vi "Read.vi"(8 "error in":errorcluster, 11 "Cycler Cluster - 24 Channel.lvclass":refnum<class "Cycler Cluster - 24 Channel.lvclass">) -> (0 "error out":errorcluster, 3 "output cluster":refnum<class "Cycler Cluster - 24 Channel.lvclass">)   [LabVIEW 2023, in "Cycler Cluster - 24 Channel.lvclass"]
uses:
  Cycler Cluster - 24 Channel.lvclass
  Cycler Cluster - 24 Channel.lvclass/Cycler Cluster - 24 Channel.ctl
  63f58f61-d796-4b25-88da-0470b2e22bf3.vi
  00f2480c-82fd-4dbd-adb2-7db79231ca1c.vi
  a45d338c-933b-4179-9ec5-1bb175e221a9.vi
  3e7895c2-778d-41f3-8bcc-0a004ba5d0e6.vi
  a5f17dcd-adde-4f08-8f4e-8c8580528fc1.vi
  ed9361c3-689c-4e9b-add1-8b87589797f0.vi
  6a4160ad-b9eb-4b5d-957b-ca1972af427b.vi
  340e8093-4c33-452f-a0fc-ec0f0c816548.vi
  4acc0959-a97e-40d2-905f-e4b53c5396e1.vi
  9ce8a87f-1424-40f7-aba3-ebfca12f9530.vi
  db8316ad-a1f6-46f4-a9d7-3ff13c7a6c53.vi
  3280034d-1119-4562-8431-d6c79152f843.vi
  5cec743d-8e0c-44d6-a509-ac96f90befc9.vi
  f015e34a-d19a-4af2-9a20-24b0ffa0b5d3.vi
  0afebac1-deb8-4dea-a382-2e4262eb9ab7.vi
  1ba67a8f-3263-44e6-b47e-6b1f46c6cf02.vi
  71f8bbf1-da11-439f-874e-3e528bdfa749.vi
  0c8128a7-c07e-44cb-ab87-c3f617b7e890.vi
  e505fce4-1dbe-4dbd-969b-5f8f6cb92da5.vi
  110d711f-602d-45bb-9c3c-bc18ca51752e.vi
  a3c512e7-962e-4a93-8488-56a803890fdd.vi
  4f6d0910-25e4-400a-b4c5-092e8cc88d34.vi
  4448cff9-e18d-4a6b-945e-10b1e3fd2828.vi
  4a46be96-aeb5-43b7-9243-adca9a8444cf.vi
  27230f32-3038-432e-846c-8983fd03581f.vi
  63f58f61-d796-4b25-88da-0470b2e22bf3.vi/c28b0ead-42ad-4072-80a2-aca7f2bd7ce3.vi
  63f58f61-d796-4b25-88da-0470b2e22bf3.vi/219d0231-d98b-4193-b5cc-84f90e3c9091.vi
  00f2480c-82fd-4dbd-adb2-7db79231ca1c.vi/c28b0ead-42ad-4072-80a2-aca7f2bd7ce3.vi
  00f2480c-82fd-4dbd-adb2-7db79231ca1c.vi/219d0231-d98b-4193-b5cc-84f90e3c9091.vi
  a45d338c-933b-4179-9ec5-1bb175e221a9.vi/c28b0ead-42ad-4072-80a2-aca7f2bd7ce3.vi
  a45d338c-933b-4179-9ec5-1bb175e221a9.vi/219d0231-d98b-4193-b5cc-84f90e3c9091.vi
  3e7895c2-778d-41f3-8bcc-0a004ba5d0e6.vi/c28b0ead-42ad-4072-80a2-aca7f2bd7ce3.vi
  3e7895c2-778d-41f3-8bcc-0a004ba5d0e6.vi/219d0231-d98b-4193-b5cc-84f90e3c9091.vi
  a5f17dcd-adde-4f08-8f4e-8c8580528fc1.vi/c28b0ead-42ad-4072-80a2-aca7f2bd7ce3.vi
  a5f17dcd-adde-4f08-8f4e-8c8580528fc1.vi/219d0231-d98b-4193-b5cc-84f90e3c9091.vi
  ed9361c3-689c-4e9b-add1-8b87589797f0.vi/c28b0ead-42ad-4072-80a2-aca7f2bd7ce3.vi
  ed9361c3-689c-4e9b-add1-8b87589797f0.vi/219d0231-d98b-4193-b5cc-84f90e3c9091.vi
  6a4160ad-b9eb-4b5d-957b-ca1972af427b.vi/c28b0ead-42ad-4072-80a2-aca7f2bd7ce3.vi
  6a4160ad-b9eb-4b5d-957b-ca1972af427b.vi/219d0231-d98b-4193-b5cc-84f90e3c9091.vi
  340e8093-4c33-452f-a0fc-ec0f0c816548.vi/c28b0ead-42ad-4072-80a2-aca7f2bd7ce3.vi
  340e8093-4c33-452f-a0fc-ec0f0c816548.vi/219d0231-d98b-4193-b5cc-84f90e3c9091.vi
  4acc0959-a97e-40d2-905f-e4b53c5396e1.vi/c28b0ead-42ad-4072-80a2-aca7f2bd7ce3.vi
  4acc0959-a97e-40d2-905f-e4b53c5396e1.vi/219d0231-d98b-4193-b5cc-84f90e3c9091.vi
  9ce8a87f-1424-40f7-aba3-ebfca12f9530.vi/c28b0ead-42ad-4072-80a2-aca7f2bd7ce3.vi
  9ce8a87f-1424-40f7-aba3-ebfca12f9530.vi/219d0231-d98b-4193-b5cc-84f90e3c9091.vi
  db8316ad-a1f6-46f4-a9d7-3ff13c7a6c53.vi/c28b0ead-42ad-4072-80a2-aca7f2bd7ce3.vi
  db8316ad-a1f6-46f4-a9d7-3ff13c7a6c53.vi/219d0231-d98b-4193-b5cc-84f90e3c9091.vi
  3280034d-1119-4562-8431-d6c79152f843.vi/c28b0ead-42ad-4072-80a2-aca7f2bd7ce3.vi
  3280034d-1119-4562-8431-d6c79152f843.vi/219d0231-d98b-4193-b5cc-84f90e3c9091.vi
  5cec743d-8e0c-44d6-a509-ac96f90befc9.vi/c28b0ead-42ad-4072-80a2-aca7f2bd7ce3.vi
  5cec743d-8e0c-44d6-a509-ac96f90befc9.vi/219d0231-d98b-4193-b5cc-84f90e3c9091.vi
  f015e34a-d19a-4af2-9a20-24b0ffa0b5d3.vi/c28b0ead-42ad-4072-80a2-aca7f2bd7ce3.vi
  f015e34a-d19a-4af2-9a20-24b0ffa0b5d3.vi/219d0231-d98b-4193-b5cc-84f90e3c9091.vi
  0afebac1-deb8-4dea-a382-2e4262eb9ab7.vi/c28b0ead-42ad-4072-80a2-aca7f2bd7ce3.vi
  0afebac1-deb8-4dea-a382-2e4262eb9ab7.vi/219d0231-d98b-4193-b5cc-84f90e3c9091.vi
  1ba67a8f-3263-44e6-b47e-6b1f46c6cf02.vi/c28b0ead-42ad-4072-80a2-aca7f2bd7ce3.vi
  1ba67a8f-3263-44e6-b47e-6b1f46c6cf02.vi/219d0231-d98b-4193-b5cc-84f90e3c9091.vi
  71f8bbf1-da11-439f-874e-3e528bdfa749.vi/c28b0ead-42ad-4072-80a2-aca7f2bd7ce3.vi
  71f8bbf1-da11-439f-874e-3e528bdfa749.vi/219d0231-d98b-4193-b5cc-84f90e3c9091.vi
  0c8128a7-c07e-44cb-ab87-c3f617b7e890.vi/c28b0ead-42ad-4072-80a2-aca7f2bd7ce3.vi
  0c8128a7-c07e-44cb-ab87-c3f617b7e890.vi/219d0231-d98b-4193-b5cc-84f90e3c9091.vi
  e505fce4-1dbe-4dbd-969b-5f8f6cb92da5.vi/c28b0ead-42ad-4072-80a2-aca7f2bd7ce3.vi
  e505fce4-1dbe-4dbd-969b-5f8f6cb92da5.vi/219d0231-d98b-4193-b5cc-84f90e3c9091.vi
  110d711f-602d-45bb-9c3c-bc18ca51752e.vi/c28b0ead-42ad-4072-80a2-aca7f2bd7ce3.vi
  110d711f-602d-45bb-9c3c-bc18ca51752e.vi/219d0231-d98b-4193-b5cc-84f90e3c9091.vi
  a3c512e7-962e-4a93-8488-56a803890fdd.vi/c28b0ead-42ad-4072-80a2-aca7f2bd7ce3.vi
  a3c512e7-962e-4a93-8488-56a803890fdd.vi/219d0231-d98b-4193-b5cc-84f90e3c9091.vi
  4f6d0910-25e4-400a-b4c5-092e8cc88d34.vi/c28b0ead-42ad-4072-80a2-aca7f2bd7ce3.vi
  4f6d0910-25e4-400a-b4c5-092e8cc88d34.vi/219d0231-d98b-4193-b5cc-84f90e3c9091.vi
  4448cff9-e18d-4a6b-945e-10b1e3fd2828.vi/c28b0ead-42ad-4072-80a2-aca7f2bd7ce3.vi
  4448cff9-e18d-4a6b-945e-10b1e3fd2828.vi/219d0231-d98b-4193-b5cc-84f90e3c9091.vi
  4a46be96-aeb5-43b7-9243-adca9a8444cf.vi/c28b0ead-42ad-4072-80a2-aca7f2bd7ce3.vi
  4a46be96-aeb5-43b7-9243-adca9a8444cf.vi/219d0231-d98b-4193-b5cc-84f90e3c9091.vi
  27230f32-3038-432e-846c-8983fd03581f.vi/c28b0ead-42ad-4072-80a2-aca7f2bd7ce3.vi
  27230f32-3038-432e-846c-8983fd03581f.vi/219d0231-d98b-4193-b5cc-84f90e3c9091.vi
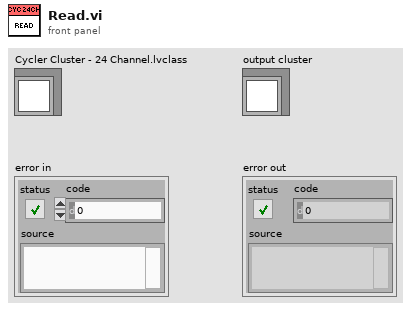
[diagram p1: front panel]
types:
  T1 = cluster{"OnOff.ACT":bool, "ErrorAcknowledge.ACT":bool, "IsoMeasurement.ACT":bool, "ParallelMode.ACT":bool}
  T2 = cluster{"ErrorAcknowledge.ch01.ACT":bool, "OutputEnable.ch01.ACT":bool, "ControlMode.ch01.CTL":u16, "Voltage.ch01.SP":dbl, "VoltageMIN.ch01.SP":dbl, "VoltageMAX.ch01.SP":dbl, "VoltageGrad.ch01.SP":dbl, "Current.ch01.SP":dbl, "CurrentMIN.ch01.SP":dbl, "CurrentMAX.ch01.SP":dbl, "CurrentGrad.ch01.SP":dbl, "Power.ch01.SP":dbl, "Power.ch01.SP":dbl, "Power.ch01.SP":dbl, "PowerGrad.ch01.SP":dbl, "ParameterSet.ch01.CTL":i32}
  T3 = cluster{"ErrorAcknowledge.ch02.ACT":bool, "OutputEnable.ch02.ACT":bool, "ControlMode.ch02.CTL":u16, "Voltage.ch02.SP":dbl, "VoltageMIN.ch02.SP":dbl, "VoltageMAX.ch02.SP":dbl, "VoltageGrad.ch02.SP":dbl, "Current.ch02.SP":dbl, "CurrentMIN.ch02.SP":dbl, "CurrentMAX.ch02.SP":dbl, "CurrentGrad.ch02.SP":dbl, "Power.ch02.SP":dbl, "PowerMIN.ch02.SP":dbl, "PowerMAX.ch02.SP":dbl, "PowerGrad.ch02.SP":dbl, "ParameterSet.ch02.CTL":i32}
  T4 = cluster{"ErrorAcknowledge.ch03.ACT":bool, "OutputEnable.ch03.ACT":bool, "ControlMode.ch03.CTL":u16, "Voltage.ch03.SP":dbl, "VoltageMIN.ch03.SP":dbl, "VoltageMAX.ch03.SP":dbl, "VoltageGrad.ch03.SP":dbl, "Current.ch03.SP":dbl, "CurrentMIN.ch03.SP":dbl, "CurrentMAX.ch03.SP":dbl, "CurrentGrad.ch03.SP":dbl, "Power.ch03.SP":dbl, "PowerMIN.ch03.SP":dbl, "PowerMAX.ch03.SP":dbl, "PowerGrad.ch03.SP":dbl, "ParameterSet.ch03.CTL":i32}
  T5 = cluster{"ErrorAcknowledge.ch04.ACT":bool, "OutputEnable.ch04.ACT":bool, "ControlMode.ch04.CTL":u16, "Voltage.ch04.SP":dbl, "VoltageMIN.ch04.SP":dbl, "VoltageMAX.ch04.SP":dbl, "VoltageGrad.ch04.SP":dbl, "Current.ch04.SP":dbl, "CurrentMIN.ch04.SP":dbl, "CurrentMAX.ch04.SP":dbl, "CurrentGrad.ch04.SP":dbl, "Power.ch04.SP":dbl, "PowerMIN.ch04.SP":dbl, "PowerMAX.ch04.SP":dbl, "PowerGrad.ch04.SP":dbl, "ParameterSet.ch04.CTL":i32}
  T6 = cluster{"ErrorAcknowledge.ch05.ACT":bool, "OutputEnable.ch05.ACT":bool, "ControlMode.ch05.CTL":u16, "Voltage.ch05.SP":dbl, "VoltageMIN.ch05.SP":dbl, "VoltageMAX.ch05.SP":dbl, "VoltageGrad.ch05.SP":dbl, "Current.ch05.SP":dbl, "CurrentMIN.ch05.SP":dbl, "CurrentMAX.ch05.SP":dbl, "CurrentGrad.ch05.SP":dbl, "Power.ch05.SP":dbl, "PowerMIN.ch05.SP":dbl, "PowerMAX.ch05.SP":dbl, "PowerGrad.ch05.SP":dbl, "ParameterSet.ch05.CTL":i32}
  T7 = cluster{"ErrorAcknowledge.ch06.ACT":bool, "OutputEnable.ch06.ACT":bool, "ControlMode.ch06.CTL":u16, "Voltage.ch06.SP":dbl, "VoltageMIN.ch06.SP":dbl, "VoltageMAX.ch06.SP":dbl, "VoltageGrad.ch06.SP":dbl, "Current.ch06.SP":dbl, "CurrentMIN.ch06.SP":dbl, "CurrentMAX.ch06.SP":dbl, "CurrentGrad.ch06.SP":dbl, "Power.ch06.SP":dbl, "PowerMIN.ch06.SP":dbl, "PowerMAX.ch06.SP":dbl, "PowerGrad.ch06.SP":dbl, "ParameterSet.ch06.CTL":i32}
  T8 = cluster{"ErrorAcknowledge.ch07.ACT":bool, "OutputEnable.ch07.ACT":bool, "ControlMode.ch07.CTL":u16, "Voltage.ch07.SP":dbl, "VoltageMIN.ch07.SP":dbl, "VoltageMAX.ch07.SP":dbl, "VoltageGrad.ch07.SP":dbl, "Current.ch07.SP":dbl, "CurrentMIN.ch07.SP":dbl, "CurrentMAX.ch07.SP":dbl, "CurrentGrad.ch07.SP":dbl, "Power.ch07.SP":dbl, "PowerMIN.ch07.SP":dbl, "PowerMAX.ch07.SP":dbl, "PowerGrad.ch07.SP":dbl, "ParameterSet.ch07.CTL":i32}
  T9 = cluster{"ErrorAcknowledge.ch08.ACT":bool, "OutputEnable.ch08.ACT":bool, "ControlMode.ch08.CTL":u16, "Voltage.ch08.SP":dbl, "VoltageMIN.ch08.SP":dbl, "VoltageMAX.ch08.SP":dbl, "VoltageGrad.ch08.SP":dbl, "Current.ch08.SP":dbl, "CurrentMIN.ch08.SP":dbl, "CurrentMAX.ch08.SP":dbl, "CurrentGrad.ch08.SP":dbl, "Power.ch08.SP":dbl, "PowerMIN.ch08.SP":dbl, "PowerMAX.ch08.SP":dbl, "PowerGrad.ch08.SP":dbl, "ParameterSet.ch08.CTL":i32}
  T10 = cluster{"ErrorAcknowledge.ch09.ACT":bool, "OutputEnable.ch09.ACT":bool, "ControlMode.ch09.CTL":u16, "Voltage.ch09.SP":dbl, "VoltageMIN.ch09.SP":dbl, "VoltageMAX.ch09.SP":dbl, "VoltageGrad.ch09.SP":dbl, "Current.ch09.SP":dbl, "CurrentMIN.ch09.SP":dbl, "CurrentMAX.ch09.SP":dbl, "CurrentGrad.ch09.SP":dbl, "Power.ch09.SP":dbl, "PowerMIN.ch09.SP":dbl, "PowerMAX.ch09.SP":dbl, "PowerGrad.ch09.SP":dbl, "ParameterSet.ch09.CTL":i32}
  T11 = cluster{"ErrorAcknowledge.ch10.ACT":bool, "OutputEnable.ch10.ACT":bool, "ControlMode.ch10.CTL":u16, "Voltage.ch10.SP":dbl, "VoltageMIN.ch10.SP":dbl, "VoltageMAX.ch10.SP":dbl, "VoltageGrad.ch10.SP":dbl, "Current.ch10.SP":dbl, "CurrentMIN.ch10.SP":dbl, "CurrentMAX.ch10.SP":dbl, "CurrentGrad.ch10.SP":dbl, "Power.ch10.SP":dbl, "PowerMIN.ch10.SP":dbl, "PowerMAX.ch10.SP":dbl, "PowerGrad.ch10.SP":dbl, "ParameterSet.ch10.CTL":i32}
  T12 = cluster{"ErrorAcknowledge.ch11.ACT":bool, "OutputEnable.ch11.ACT":bool, "ControlMode.ch11.CTL":u16, "Voltage.ch11.SP":dbl, "VoltageMIN.ch11.SP":dbl, "VoltageMAX.ch11.SP":dbl, "VoltageGrad.ch11.SP":dbl, "Current.ch11.SP":dbl, "CurrentMIN.ch11.SP":dbl, "CurrentMAX.ch11.SP":dbl, "CurrentGrad.ch11.SP":dbl, "Power.ch11.SP":dbl, "PowerMIN.ch11.SP":dbl, "PowerMAX.ch11.SP":dbl, "PowerGrad.ch11.SP":dbl, "ParameterSet.ch11.CTL":i32}
  T13 = cluster{"ErrorAcknowledge.ch12.ACT":bool, "OutputEnable.ch12.ACT":bool, "ControlMode.ch12.CTL":u16, "Voltage.ch12.SP":dbl, "VoltageMIN.ch12.SP":dbl, "VoltageMAX.ch12.SP":dbl, "VoltageGrad.ch12.SP":dbl, "Current.ch12.SP":dbl, "CurrentMIN.ch12.SP":dbl, "CurrentMAX.ch12.SP":dbl, "CurrentGrad.ch12.SP":dbl, "Power.ch12.SP":dbl, "PowerMIN.ch12.SP":dbl, "PowerMAX.ch12.SP":dbl, "PowerGrad.ch12.SP":dbl, "ParameterSet.ch12.CTL":i32}
  T14 = cluster{"ErrorAcknowledge.ch13.ACT":bool, "OutputEnable.ch13.ACT":bool, "ControlMode.ch13.CTL":u16, "Voltage.ch13.SP":dbl, "VoltageMIN.ch13.SP":dbl, "VoltageMAX.ch13.SP":dbl, "VoltageGrad.ch13.SP":dbl, "Current.ch13.SP":dbl, "CurrentMIN.ch13.SP":dbl, "CurrentMAX.ch13.SP":dbl, "CurrentGrad.ch13.SP":dbl, "Power.ch13.SP":dbl, "PowerMIN.ch13.SP":dbl, "PowerMAX.ch13.SP":dbl, "PowerGrad.ch13.SP":dbl, "ParameterSet.ch13.CTL":i32}
  T15 = cluster{"ErrorAcknowledge.ch14.ACT":bool, "OutputEnable.ch14.ACT":bool, "ControlMode.ch14.CTL":u16, "Voltage.ch14.SP":dbl, "VoltageMIN.ch14.SP":dbl, "VoltageMAX.ch14.SP":dbl, "VoltageGrad.ch14.SP":dbl, "Current.ch14.SP":dbl, "CurrentMIN.ch14.SP":dbl, "CurrentMAX.ch14.SP":dbl, "CurrentGrad.ch14.SP":dbl, "Power.ch14.SP":dbl, "PowerMIN.ch14.SP":dbl, "PowerMAX.ch14.SP":dbl, "PowerGrad.ch14.SP":dbl, "ParameterSet.ch14.CTL":i32}
  T16 = cluster{"ErrorAcknowledge.ch15.ACT":bool, "OutputEnable.ch15.ACT":bool, "ControlMode.ch15.CTL":u16, "Voltage.ch15.SP":dbl, "VoltageMIN.ch15.SP":dbl, "VoltageMAX.ch15.SP":dbl, "VoltageGrad.ch15.SP":dbl, "Current.ch15.SP":dbl, "CurrentMIN.ch15.SP":dbl, "CurrentMAX.ch15.SP":dbl, "CurrentGrad.ch15.SP":dbl, "Power.ch15.SP":dbl, "PowerMIN.ch15.SP":dbl, "PowerMAX.ch15.SP":dbl, "PowerGrad.ch15.SP":dbl, "ParameterSet.ch15.CTL":i32}
  T17 = cluster{"ErrorAcknowledge.ch16.ACT":bool, "OutputEnable.ch16.ACT":bool, "ControlMode.ch16.CTL":u16, "Voltage.ch16.SP":dbl, "VoltageMIN.ch16.SP":dbl, "VoltageMAX.ch16.SP":dbl, "VoltageGrad.ch16.SP":dbl, "Current.ch16.SP":dbl, "CurrentMIN.ch16.SP":dbl, "CurrentMAX.ch16.SP":dbl, "CurrentGrad.ch16.SP":dbl, "Power.ch16.SP":dbl, "PowerMIN.ch16.SP":dbl, "PowerMAX.ch16.SP":dbl, "PowerGrad.ch16.SP":dbl, "ParameterSet.ch16.CTL":i32}
  T18 = cluster{"ErrorAcknowledge.ch17.ACT":bool, "OutputEnable.ch17.ACT":bool, "ControlMode.ch17.CTL":u16, "Voltage.ch17.SP":dbl, "VoltageMIN.ch17.SP":dbl, "VoltageMAX.ch17.SP":dbl, "VoltageGrad.ch17.SP":dbl, "Current.ch17.SP":dbl, "CurrentMIN.ch17.SP":dbl, "CurrentMAX.ch17.SP":dbl, "CurrentGrad.ch17.SP":dbl, "Power.ch17.SP":dbl, "PowerMIN.ch17.SP":dbl, "PowerMAX.ch17.SP":dbl, "PowerGrad.ch17.SP":dbl, "ParameterSet.ch17.CTL":i32}
  T19 = cluster{"ErrorAcknowledge.ch18.ACT":bool, "OutputEnable.ch18.ACT":bool, "ControlMode.ch18.CTL":u16, "Voltage.ch18.SP":dbl, "VoltageMIN.ch18.SP":dbl, "VoltageMAX.ch18.SP":dbl, "VoltageGrad.ch18.SP":dbl, "Current.ch18.SP":dbl, "CurrentMIN.ch18.SP":dbl, "CurrentMAX.ch18.SP":dbl, "CurrentGrad.ch18.SP":dbl, "Power.ch18.SP":dbl, "PowerMIN.ch18.SP":dbl, "PowerMAX.ch18.SP":dbl, "PowerGrad.ch18.SP":dbl, "ParameterSet.ch18.CTL":i32}
  T20 = cluster{"ErrorAcknowledge.ch19.ACT":bool, "OutputEnable.ch19.ACT":bool, "ControlMode.ch19.CTL":u16, "Voltage.ch19.SP":dbl, "VoltageMIN.ch19.SP":dbl, "VoltageMAX.ch19.SP":dbl, "VoltageGrad.ch19.SP":dbl, "Current.ch19.SP":dbl, "CurrentMIN.ch19.SP":dbl, "CurrentMAX.ch19.SP":dbl, "CurrentGrad.ch19.SP":dbl, "Power.ch19.SP":dbl, "PowerMIN.ch19.SP":dbl, "PowerMAX.ch19.SP":dbl, "PowerGrad.ch19.SP":dbl, "ParameterSet.ch19.CTL":i32}
  T21 = cluster{"ErrorAcknowledge.ch20.ACT":bool, "OutputEnable.ch20.ACT":bool, "ControlMode.ch20.CTL":u16, "Voltage.ch20.SP":dbl, "VoltageMIN.ch20.SP":dbl, "VoltageMAX.ch20.SP":dbl, "VoltageGrad.ch20.SP":dbl, "Current.ch20.SP":dbl, "CurrentMIN.ch20.SP":dbl, "CurrentMAX.ch20.SP":dbl, "CurrentGrad.ch20.SP":dbl, "Power.ch20.SP":dbl, "PowerMIN.ch20.SP":dbl, "PowerMAX.ch20.SP":dbl, "PowerGrad.ch20.SP":dbl, "ParameterSet.ch20.CTL":i32}
  T22 = cluster{"ErrorAcknowledge.ch21.ACT":bool, "OutputEnable.ch21.ACT":bool, "ControlMode.ch21.CTL":u16, "Voltage.ch21.SP":dbl, "VoltageMIN.ch21.SP":dbl, "VoltageMAX.ch21.SP":dbl, "VoltageGrad.ch21.SP":dbl, "Current.ch21.SP":dbl, "CurrentMIN.ch21.SP":dbl, "CurrentMAX.ch21.SP":dbl, "CurrentGrad.ch21.SP":dbl, "Power.ch21.SP":dbl, "PowerMIN.ch21.SP":dbl, "PowerMAX.ch21.SP":dbl, "PowerGrad.ch21.SP":dbl, "ParameterSet.ch21.CTL":i32}
  T23 = cluster{"ErrorAcknowledge.ch22.ACT":bool, "OutputEnable.ch22.ACT":bool, "ControlMode.ch22.CTL":u16, "Voltage.ch22.SP":dbl, "VoltageMIN.ch22.SP":dbl, "VoltageMAX.ch22.SP":dbl, "VoltageGrad.ch22.SP":dbl, "Current.ch22.SP":dbl, "CurrentMIN.ch22.SP":dbl, "CurrentMAX.ch22.SP":dbl, "CurrentGrad.ch22.SP":dbl, "Power.ch22.SP":dbl, "PowerMIN.ch22.SP":dbl, "PowerMAX.ch22.SP":dbl, "PowerGrad.ch22.SP":dbl, "ParameterSet.ch22.CTL":i32}
  T24 = cluster{"ErrorAcknowledge.ch23.ACT":bool, "OutputEnable.ch23.ACT":bool, "ControlMode.ch23.CTL":u16, "Voltage.ch23.SP":dbl, "VoltageMIN.ch23.SP":dbl, "VoltageMAX.ch23.SP":dbl, "VoltageGrad.ch23.SP":dbl, "Current.ch23.SP":dbl, "CurrentMIN.ch23.SP":dbl, "CurrentMAX.ch23.SP":dbl, "CurrentGrad.ch23.SP":dbl, "Power.ch23.SP":dbl, "PowerMIN.ch23.SP":dbl, "PowerMAX.ch23.SP":dbl, "PowerGrad.ch23.SP":dbl, "ParameterSet.ch23.CTL":i32}
  T25 = cluster{"ErrorAcknowledge.ch24.ACT":bool, "OutputEnable.ch24.ACT":bool, "ControlMode.ch24.CTL":u16, "Voltage.ch24.SP":dbl, "VoltageMIN.ch24.SP":dbl, "VoltageMAX.ch24.SP":dbl, "VoltageGrad.ch24.SP":dbl, "Current.ch24.SP":dbl, "CurrentMIN.ch24.SP":dbl, "CurrentMAX.ch24.SP":dbl, "CurrentGrad.ch24.SP":dbl, "Power.ch24.SP":dbl, "PowerMIN.ch24.SP":dbl, "PowerMAX.ch24.SP":dbl, "PowerGrad.ch24.SP":dbl, "ParameterSet.ch24.CTL":i32}
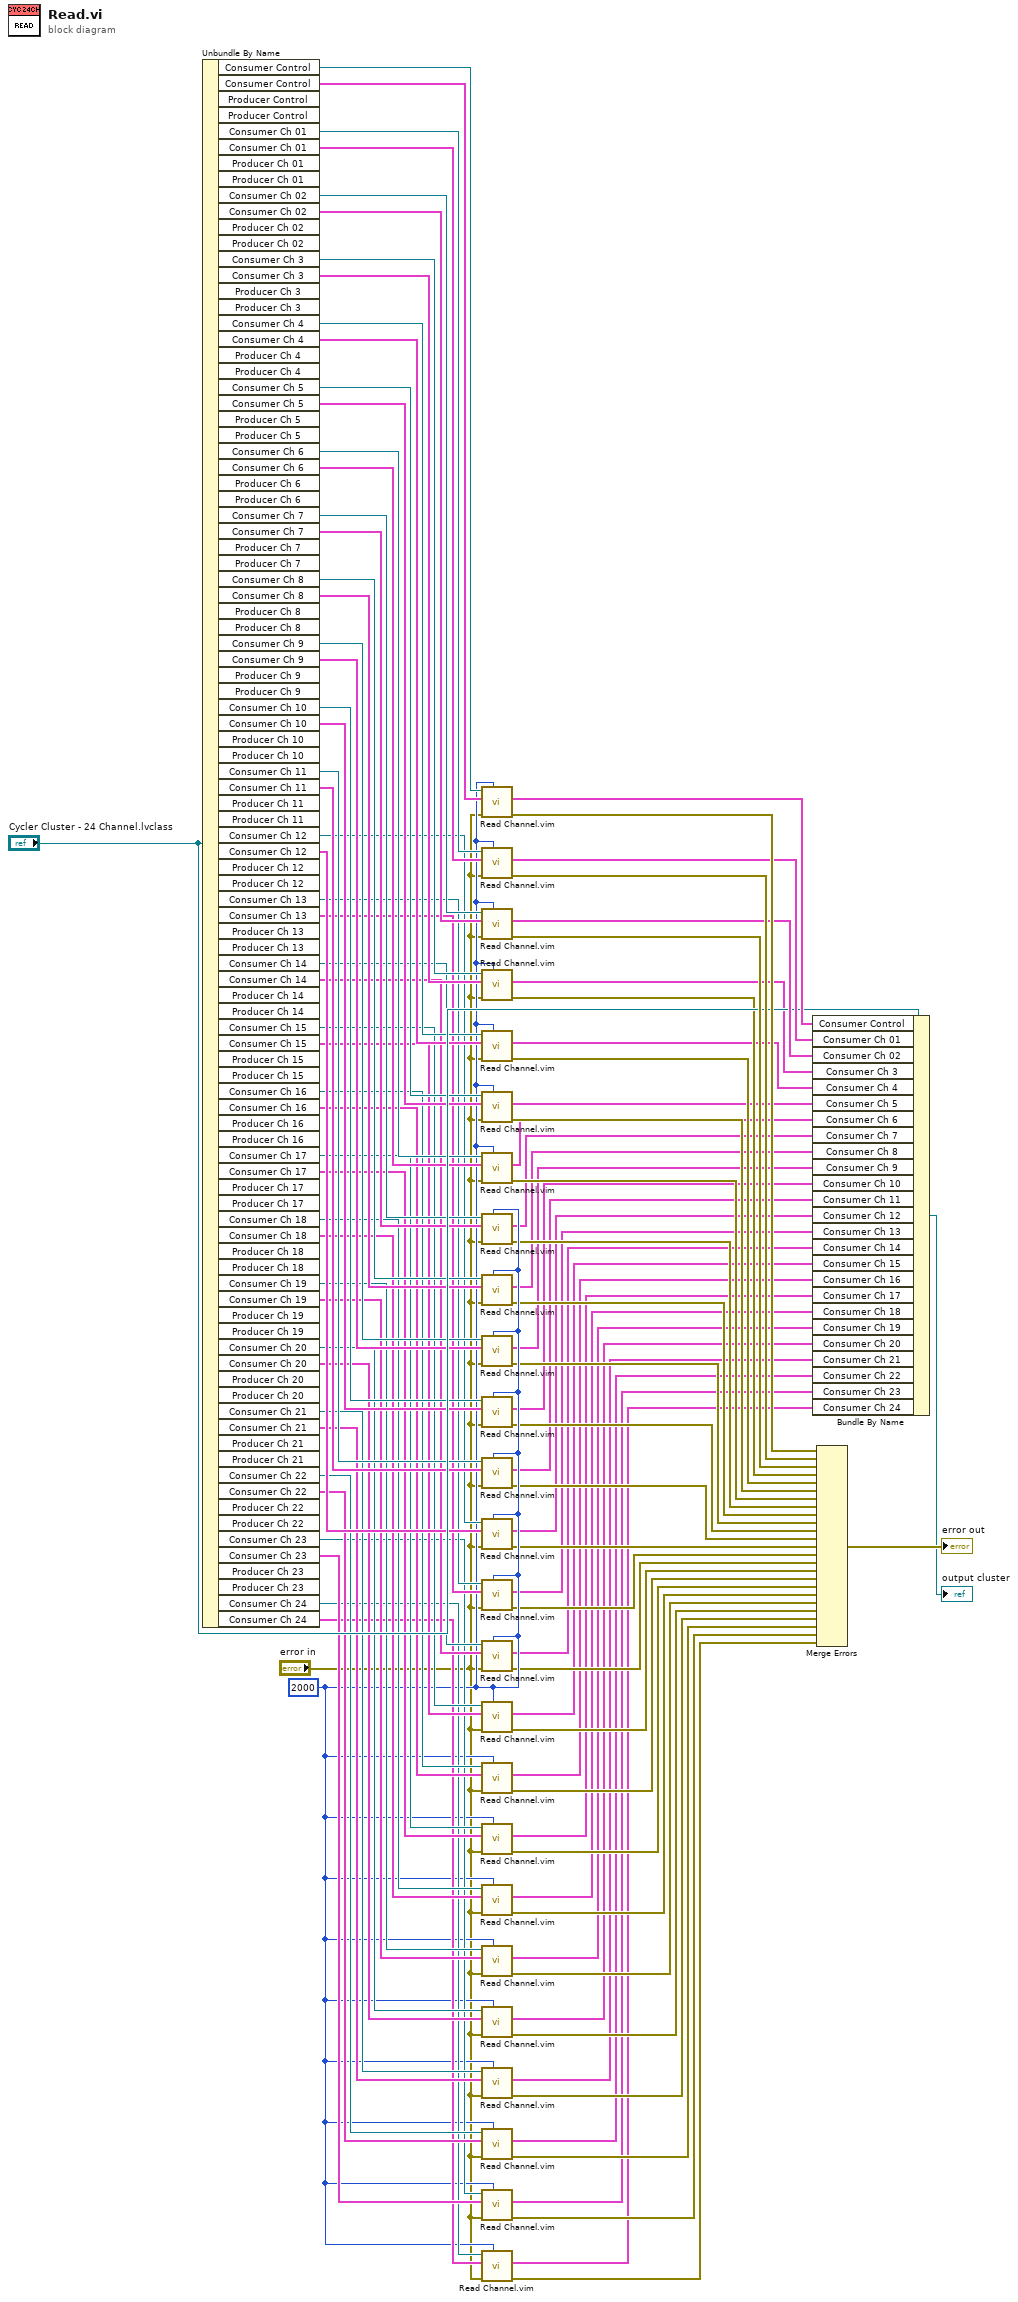
[diagram p0: block diagram]
diagram:
  w46 = 2000 ("Timeout (ms)")
  n1 = Unbundle By Name("Cycler Cluster - 24 Channel.lvclass") -> ("Consumer Control"=w96:refnum<k21>, "Consumer Control"=w95:T1, "Consumer Ch 01"=w94:refnum<k21>, "Consumer Ch 01"=w93:T2, "Consumer Ch 02"=w92:refnum<k21>, "Consumer Ch 02"=w91:T3, "Consumer Ch 3"=w90:refnum<k21>, "Consumer Ch 3"=w89:T4, "Consumer Ch 4"=w88:refnum<k21>, "Consumer Ch 4"=w87:T5, "Consumer Ch 5"=w86:refnum<k21>, "Consumer Ch 5"=w85:T6, "Consumer Ch 6"=w84:refnum<k21>, "Consumer Ch 6"=w83:T7, "Consumer Ch 7"=w82:refnum<k21>, "Consumer Ch 7"=w81:T8, "Consumer Ch 8"=w80:refnum<k21>, "Consumer Ch 8"=w79:T9, "Consumer Ch 9"=w78:refnum<k21>, "Consumer Ch 9"=w77:T10, "Consumer Ch 10"=w76:refnum<k21>, "Consumer Ch 10"=w75:T11, "Consumer Ch 11"=w74:refnum<k21>, "Consumer Ch 11"=w73:T12, "Consumer Ch 12"=w72:refnum<k21>, "Consumer Ch 12"=w71:T13, "Consumer Ch 13"=w70:refnum<k21>, "Consumer Ch 13"=w69:T14, "Consumer Ch 14"=w68:refnum<k21>, "Consumer Ch 14"=w67:T15, "Consumer Ch 15"=w66:refnum<k21>, "Consumer Ch 15"=w65:T16, "Consumer Ch 16"=w64:refnum<k21>, "Consumer Ch 16"=w63:T17, "Consumer Ch 17"=w62:refnum<k21>, "Consumer Ch 17"=w61:T18, "Consumer Ch 18"=w60:refnum<k21>, "Consumer Ch 18"=w59:T19, "Consumer Ch 19"=w58:refnum<k21>, "Consumer Ch 19"=w57:T20, "Consumer Ch 20"=w56:refnum<k21>, "Consumer Ch 20"=w55:T21, "Consumer Ch 21"=w54:refnum<k21>, "Consumer Ch 21"=w53:T22, "Consumer Ch 22"=w52:refnum<k21>, "Consumer Ch 22"=w51:T23, "Consumer Ch 23"=w50:refnum<k21>, "Consumer Ch 23"=w49:T24, "Consumer Ch 24"=w48:refnum<k21>, "Consumer Ch 24"=w47:T25)  [unwired: 48 out]
  n2 = call "Read Channel.vim"("Timeout (ms)"=w46, "error in"="error in", "Data in"=w95, "ADAS HIL Channel in"=w96) -> ("error out"=w104:errorcluster, "Data out"=w105:T1)  [unwired: 4 in, 2 out]
  n3 = call "Read Channel.vim"("Timeout (ms)"=w46, "error in"="error in", "Data in"=w93, "ADAS HIL Channel in"=w94) -> ("error out"=w103:errorcluster, "Data out"=w101:T2)  [unwired: 4 in, 2 out]
  n4 = call "Read Channel.vim"("Timeout (ms)"=w46, "error in"="error in", "Data in"=w91, "ADAS HIL Channel in"=w92) -> ("error out"=w100:errorcluster, "Data out"=w99:T3)  [unwired: 4 in, 2 out]
  n5 = call "Read Channel.vim"("Timeout (ms)"=w46, "error in"="error in", "Data in"=w89, "ADAS HIL Channel in"=w90) -> ("error out"=w44:errorcluster, "Data out"=w22:T4)  [unwired: 4 in, 2 out]
  n6 = call "Read Channel.vim"("Timeout (ms)"=w46, "error in"="error in", "Data in"=w87, "ADAS HIL Channel in"=w88) -> ("error out"=w43:errorcluster, "Data out"=w21:T5)  [unwired: 4 in, 2 out]
  n7 = call "Read Channel.vim"("Timeout (ms)"=w46, "error in"="error in", "Data in"=w85, "ADAS HIL Channel in"=w86) -> ("error out"=w42:errorcluster, "Data out"=w20:T6)  [unwired: 4 in, 2 out]
  n8 = call "Read Channel.vim"("Timeout (ms)"=w46, "error in"="error in", "Data in"=w83, "ADAS HIL Channel in"=w84) -> ("error out"=w41:errorcluster, "Data out"=w19:T7)  [unwired: 4 in, 2 out]
  n9 = call "Read Channel.vim"("Timeout (ms)"=w46, "error in"="error in", "Data in"=w81, "ADAS HIL Channel in"=w82) -> ("error out"=w40:errorcluster, "Data out"=w18:T8)  [unwired: 4 in, 2 out]
  n10 = call "Read Channel.vim"("Timeout (ms)"=w46, "error in"="error in", "Data in"=w79, "ADAS HIL Channel in"=w80) -> ("error out"=w39:errorcluster, "Data out"=w17:T9)  [unwired: 4 in, 2 out]
  n11 = call "Read Channel.vim"("Timeout (ms)"=w46, "error in"="error in", "Data in"=w77, "ADAS HIL Channel in"=w78) -> ("error out"=w38:errorcluster, "Data out"=w16:T10)  [unwired: 4 in, 2 out]
  n12 = call "Read Channel.vim"("Timeout (ms)"=w46, "error in"="error in", "Data in"=w75, "ADAS HIL Channel in"=w76) -> ("error out"=w37:errorcluster, "Data out"=w15:T11)  [unwired: 4 in, 2 out]
  n13 = call "Read Channel.vim"("Timeout (ms)"=w46, "error in"="error in", "Data in"=w73, "ADAS HIL Channel in"=w74) -> ("error out"=w36:errorcluster, "Data out"=w14:T12)  [unwired: 4 in, 2 out]
  n14 = call "Read Channel.vim"("Timeout (ms)"=w46, "error in"="error in", "Data in"=w71, "ADAS HIL Channel in"=w72) -> ("error out"=w35:errorcluster, "Data out"=w13:T13)  [unwired: 4 in, 2 out]
  n15 = call "Read Channel.vim"("Timeout (ms)"=w46, "error in"="error in", "Data in"=w69, "ADAS HIL Channel in"=w70) -> ("error out"=w34:errorcluster, "Data out"=w12:T14)  [unwired: 4 in, 2 out]
  n16 = call "Read Channel.vim"("Timeout (ms)"=w46, "error in"="error in", "Data in"=w67, "ADAS HIL Channel in"=w68) -> ("error out"=w33:errorcluster, "Data out"=w11:T15)  [unwired: 4 in, 2 out]
  n17 = call "Read Channel.vim"("Timeout (ms)"=w46, "error in"="error in", "Data in"=w65, "ADAS HIL Channel in"=w66) -> ("error out"=w32:errorcluster, "Data out"=w10:T16)  [unwired: 4 in, 2 out]
  n18 = call "Read Channel.vim"("Timeout (ms)"=w46, "error in"="error in", "Data in"=w63, "ADAS HIL Channel in"=w64) -> ("error out"=w31:errorcluster, "Data out"=w9:T17)  [unwired: 4 in, 2 out]
  n19 = call "Read Channel.vim"("Timeout (ms)"=w46, "error in"="error in", "Data in"=w61, "ADAS HIL Channel in"=w62) -> ("error out"=w30:errorcluster, "Data out"=w8:T18)  [unwired: 4 in, 2 out]
  n20 = call "Read Channel.vim"("Timeout (ms)"=w46, "error in"="error in", "Data in"=w59, "ADAS HIL Channel in"=w60) -> ("error out"=w29:errorcluster, "Data out"=w7:T19)  [unwired: 4 in, 2 out]
  n21 = call "Read Channel.vim"("Timeout (ms)"=w46, "error in"="error in", "Data in"=w57, "ADAS HIL Channel in"=w58) -> ("error out"=w28:errorcluster, "Data out"=w6:T20)  [unwired: 4 in, 2 out]
  n22 = call "Read Channel.vim"("Timeout (ms)"=w46, "error in"="error in", "Data in"=w55, "ADAS HIL Channel in"=w56) -> ("error out"=w27:errorcluster, "Data out"=w5:T21)  [unwired: 4 in, 2 out]
  n23 = call "Read Channel.vim"("Timeout (ms)"=w46, "error in"="error in", "Data in"=w53, "ADAS HIL Channel in"=w54) -> ("error out"=w26:errorcluster, "Data out"=w4:T22)  [unwired: 4 in, 2 out]
  n24 = call "Read Channel.vim"("Timeout (ms)"=w46, "error in"="error in", "Data in"=w51, "ADAS HIL Channel in"=w52) -> ("error out"=w25:errorcluster, "Data out"=w3:T23)  [unwired: 4 in, 2 out]
  n25 = call "Read Channel.vim"("Timeout (ms)"=w46, "error in"="error in", "Data in"=w49, "ADAS HIL Channel in"=w50) -> ("error out"=w24:errorcluster, "Data out"=w2:T24)  [unwired: 4 in, 2 out]
  n26 = call "Read Channel.vim"("Timeout (ms)"=w46, "error in"="error in", "Data in"=w47, "ADAS HIL Channel in"=w48) -> ("error out"=w23:errorcluster, "Data out"=w1:T25)  [unwired: 4 in, 2 out]
  n27 = Bundle By Name(cluster="Cycler Cluster - 24 Channel.lvclass", "Consumer Control"=w105, "Consumer Ch 01"=w101, "Consumer Ch 02"=w99, "Consumer Ch 3"=w22, "Consumer Ch 4"=w21, "Consumer Ch 5"=w20, "Consumer Ch 6"=w19, "Consumer Ch 7"=w18, "Consumer Ch 8"=w17, "Consumer Ch 9"=w16, "Consumer Ch 10"=w15, "Consumer Ch 11"=w14, "Consumer Ch 12"=w13, "Consumer Ch 13"=w12, "Consumer Ch 14"=w11, "Consumer Ch 15"=w10, "Consumer Ch 16"=w9, "Consumer Ch 17"=w8, "Consumer Ch 18"=w7, "Consumer Ch 19"=w6, "Consumer Ch 20"=w5, "Consumer Ch 21"=w4, "Consumer Ch 22"=w3, "Consumer Ch 23"=w2, "Consumer Ch 24"=w1) -> (→"output cluster":refnum<class "Cycler Cluster - 24 Channel.lvclass">)
  n28 = Merge Errors(w104, w103, w100, w44, w43, w42, w41, w40, w39, w38, w37, w36, w35, w34, w33, w32, w31, w30, w29, w28, w27, w26, w25, w24, w23) -> (→"error out":errorcluster)
